vi "Run VI.vi"(7 "Auto Dispose Ref":bool, 8 "error in (no error)":errorcluster caption="错误输入（无错误）", 9 "Exec.State":T1(ring), 10 "clone vi?":bool, 11 "VI*":refnum<vi>) -> (0 "error out":errorcluster caption="错误输出", 3 "VI*":refnum<vi>)   [LabVIEW 2016, in "PanelDataNode.lvclass"]
uses:
  PanelDataNode.lvclass
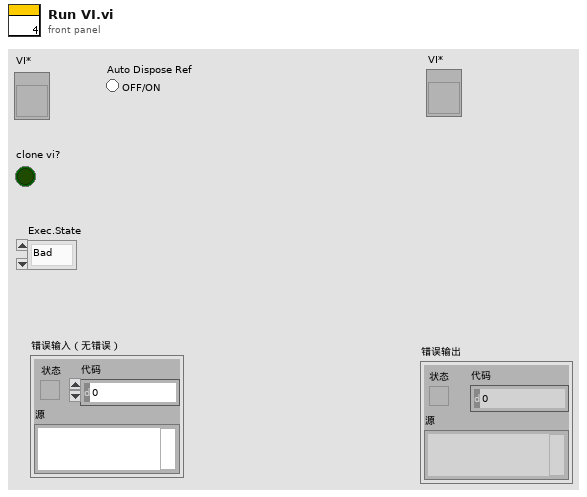
[diagram p1: front panel]
types:
  T1 = enum32{"Bad", "Idle", "Run top level", "Running"}
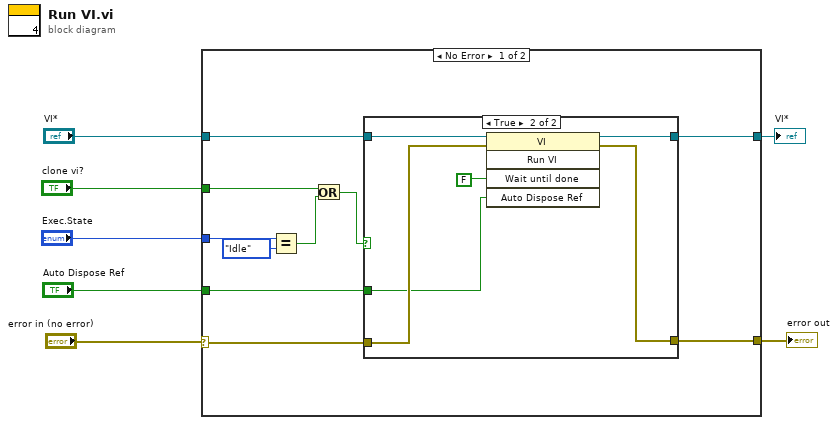
[diagram p0: block diagram]
diagram:
  n1 = case shown="No Error" "error in (no error)" {
    selector: "error in (no error)" -> [w15 w27]
    tunnel: "VI*" -> [w17 w26]
    tunnel: "clone vi?" -> [w11 _]
    tunnel: "Exec.State" -> [w16 _]
    tunnel: [w14 w27] -> w3
    tunnel: [w13 w26] -> w2
    tunnel: "Auto Dispose Ref" -> [w8 _]
    frame No Error {
      n2 = Equal?(x=w16, y=T1."Idle") -> (x = y?=w10:bool)
      n3 = Or(x=w11, y=w10) -> (x .or. y?=w9:bool)
      n4 = case shown="True" w9 {
        tunnel: w17 -> [w19 w25]
        tunnel: [w19 w23] -> w13
        tunnel: w15 -> [w18 w22]
        tunnel: [w18 w21] -> w14
        tunnel: w8 -> [_ w20]
        frame False {
        }
        frame True {
          n5 = invoke class="VI" method="Run VI"(reference=w25, error in=w22, "Wait until done"=FALSE ("结束前等待"), "Auto Dispose Ref"=w20) -> (reference out=w23:refnum<vi>, error out=w21:errorcluster)  [unwired: 1 in, 3 out]
        }
      }
    }
    frame Error {
    }
  }
  "error out" <- w3
  "VI*" <- w2
